vi "DCMotors.vi"(6 "Stop":bool, 8 "error in":errorcluster, 9 "Motors Renum":cluster{"Num":i32, "Directly":bool, "KM":dbl}[](array[cluster])=[{"Num"=1, "Directly"=TRUE, "KM"=0.97}, {"Num"=3, "Directly"=FALSE, "KM"=1.0}, {"Num"=0, "Directly"=FALSE, "KM"=0.98}, {"Num"=2, "Directly"=TRUE, "KM"=1.0}], 10 "Input":dbl[](array[slide])=[0.0, 0.0, -0.01, 0.0] step=1.0 scale=-100.0..100.0, 11 "CAN in":refnum<class "CAN.lvclass">) -> (0 "error out":errorcluster, 3 "CAN out":refnum<class "CAN.lvclass">)   [LabVIEW 2020]
uses:
  <vilib>/High Genius/HG_WSI_Tookit/Dependencies/Library/CAN/CAN.lvclass
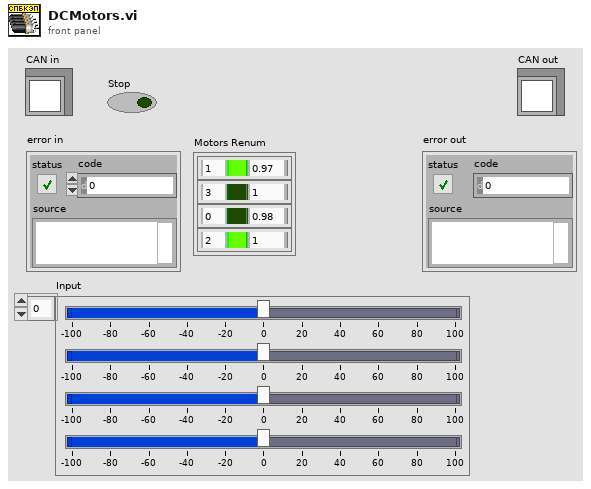
[diagram p1: front panel]
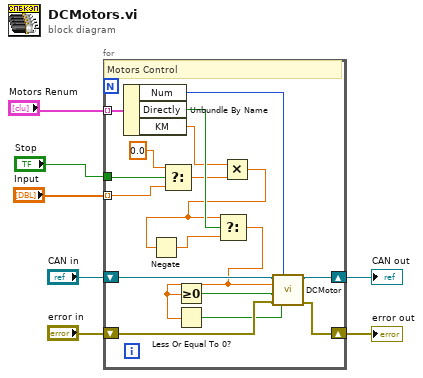
[diagram p0: block diagram]
diagram:
  n1 = for {
    shift-right: [w17] -> w6
    shift-left: "CAN in" -> [w16]
    shift-right: [w13] -> w4
    shift-left: "error in" -> [w14]
    tunnel: "Input" -> [w21] mode=indexing
    tunnel: "Motors Renum" -> [w23] mode=indexing
    tunnel: "Stop" -> [w19]
    # "Motors Control"
    n2 = Unbundle By Name(w23) -> ("Num"=w18:i32, "Directly"=w22:bool, "KM"=w8:dbl)
    n3 = Select(t=0.0, s=w19, f=w21) -> (s? t:f=w9:dbl)
    n4 = Multiply(x=w8, y=w9) -> (x*y=w10:dbl)
    n5 = Negate(x=w10) -> (-x=w24:dbl)
    n6 = Select(t=w10, s=w22, f=w24) -> (s? t:f=w11:dbl)
    n7 = Greater Or Equal To 0?(x=w11) -> (x >= 0?=w15:bool)
    n8 = Less Or Equal To 0?(x=w11) -> (x <= 0?=w12:bool)
    n9 = call "DCMotor.vi"("INB"=w12, "PWM"=w18, "error in (no error)"=w14, "INA"=w15, "Duty Cycle"=w11, "CAN in"=w16) -> ("error out"=w13:errorcluster, "CAN out"=w17:refnum<class "CAN.lvclass">)  [unwired: 4 in]
  }
  "CAN out" <- w6
  "error out" <- w4
